vi "_Raise WebMessageReceived.vi"(4 "WebView2.lvlib:WebView2 Control.lvclass":refnum<class "WebView2 Control.lvclass">, 5 "Event Data":cluster{"sender":refnum<k24>, "e":refnum<k24>}, 6 "Control Ref":refnum<k24>, 7 "Event Common Data":T1) -> ()   [LabVIEW 2025, in "WebView2.lvlib" / "WebView2 Control.lvclass"]
uses:
  WebView2 Control.lvclass
  E:/Labview/LV 2023/PPL/PPL Builder/Libs/LV-WebView2/Source/Libs/Microsoft.Web.WebView2.Core.dll
  Libs/Microsoft.Web.WebView2.Core.dll
  WebView2 Control.lvclass/WebView2 Control.ctl
  Web Message Received Event Data.ctl
  WebView2 Event Filter Interface/WebView2 Event Filter Interface.lvclass
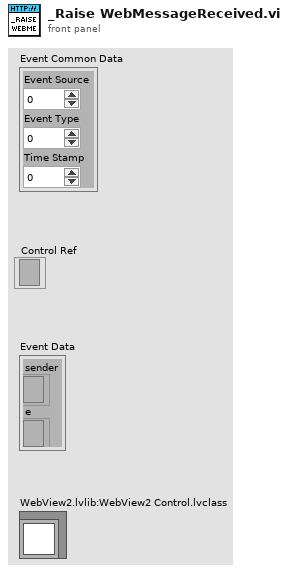
[diagram p1: front panel]
types:
  T1 = cluster{"Event Source":i32, "Event Type":u32, "Time Stamp":u32}
  T2 = typedef "WebView2.lvlib/WebView2 Control.lvclass/Web Message Received Event Data.ctl" = cluster{"Source":string, "WebMessageAsJson":string, "AdditionalObjects":refnum<k24>}
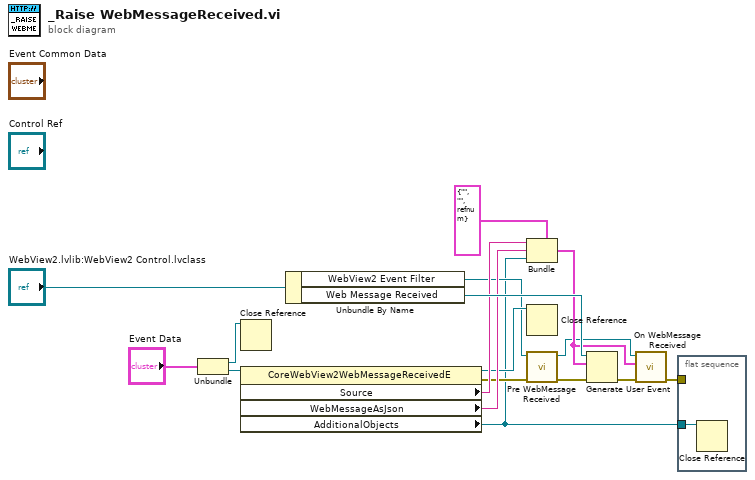
[diagram p0: block diagram]
diagram:
  n1 = Unbundle("Event Data") -> ("sender"=w11:refnum<k24>, "e"=w14:refnum<k24>)
  n2 = Close Reference(reference=w11) -> ()  [unwired: 1 in, 1 out]
  n3 = property class="CoreWebView2WebMessageReceivedE"(reference=w14) -> (reference out=w10:refnum<k24>, error out=w5:errorcluster, "Source"=w13:string, "WebMessageAsJson"=w12:string, "AdditionalObjects"=w1:refnum<k24>)  [unwired: 1 in]
  n4 = Unbundle By Name("WebView2.lvlib:WebView2 Control.lvclass") -> ("WebView2 Event Filter"=w7:refnum<class "WebView2 Event Filter Interface.lvclass">, "Web Message Received"=w15:refnum<user-event>)
  n5 = Bundle(cluster=T2 {"Source"="", "WebMessageAsJson"="", "AdditionalObjects"=refnum}, "Source"=w13, "WebMessageAsJson"=w12, "AdditionalObjects"=w1) -> (w8:T2)
  n6 = Close Reference(reference=w10) -> ()  [unwired: 1 in, 1 out]
  n7 = call-dynamic "Pre WebMessage Received.vi"("error in (no error)"=w5, "WebView2 Event Filter Interface in"=w7) -> ("error out"=w4:errorcluster, "WebView2 Event Filter Interface out"=w6:refnum<class "WebView2 Event Filter Interface.lvclass">)  [unwired: 8 in]
  n8 = Generate User Event(user event=w15, event data cluster=w8, error in=w4) -> (error out=w3:errorcluster)  [unwired: 1 in, 1 out]
  n9 = call-dynamic "On WebMessage Received.vi"("error in (no error)"=w3, "Data"=w8, "WebView2 Event Filter Interface in"=w6) -> ("error out"=w2:errorcluster)  [unwired: 7 in, 1 out]
  n10 = flat-sequence {
    tunnel: w2 -> [_]
    tunnel: w1 -> [w18]
    frame #0 {
      n11 = Close Reference(reference=w18) -> ()  [unwired: 1 in, 1 out]
    }
  }
